vi "readParameter.vi"(0 "Mockbus in":refnum<class "Mockbus.lvclass">, 5 "Input":string, 11 "error in (no error)":errorcluster) -> (4 "Mockbus out":refnum<class "Mockbus.lvclass">, 6 "Output":string, 8 "Parameter":string, 10 "LastParameter":bool, 15 "error out":errorcluster)   [LabVIEW 2015, in "RTMockbus.lvlib" / "Mockbus.lvclass"]
uses:
  Mockbus.lvclass
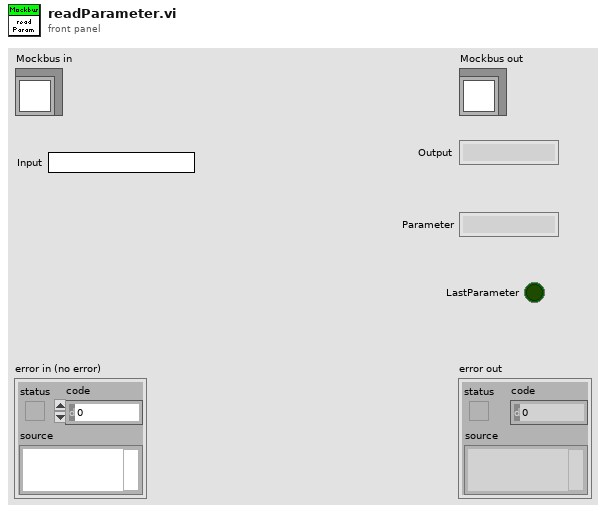
[diagram p1: front panel]
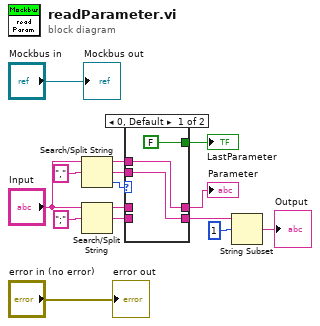
[diagram p0: block diagram]
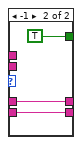
[diagram p2: hidden frame]
diagram:
  n1 = Search/Split String(string="Input", search string/char (-)=",") -> (substring before match=w11:string, match + rest of string=w10:string, offset of match=w12:i32)  [unwired: 1 in]
  n2 = Search/Split String(string="Input", search string/char (-)=";") -> (substring before match=w9:string, match + rest of string=w8:string)  [unwired: 1 in, 1 out]
  n3 = case shown="0, Default" w12 {
    tunnel: [w18 w21] -> w6
    tunnel: w11 -> [w18 _]
    tunnel: [w17 w20] -> w4
    tunnel: w10 -> [w17 _]
    tunnel: w9 -> [_ w21]
    tunnel: w8 -> [_ w20]
    tunnel: [FALSE TRUE] -> w7
    frame 0, Default {
    }
    frame -1 {
    }
  }
  "LastParameter" <- w7
  "Parameter" <- w6
  n4 = String Subset(string=w4, offset (0)=1) -> (substring=→"Output":string)  [unwired: 1 in]
  "error out" <- "error in (no error)"
  "Mockbus out" <- "Mockbus in"
